vi "FPGA Main_Scripted_OneNode_5-20-2015.vi"() -> ()   [LabVIEW 2014]
uses:
  <vilib>/rvi/Emulation/niFpgaGetClockAttributes.vi
  <vilib>/rvi/Emulation/niFpgaSctlEmulationGetInTimedLoop.vi
  <vilib>/rvi/Emulation/niFpgaEmulationReportErrorSimple.vi
  <vilib>/rvi/Emulation/niFpgaProcessEmulError.vi
  <vilib>/rvi/interface/RandomDataEmulation/niFpgaRandomDataHandleErrors.vi
  <vilib>/rvi/Emulation/niFpgaCriticalErrorInLSC.vi
  <vilib>/rvi/DataTransferAndStorage/Container/XNode/niFpgaContainer.xnode
  <vilib>/rvi/interface/RandomDataEmulation/nirviRandomDataFpgaReadWriteTemplate.vi
  SPIBus0/IO Node Logic Template_SPIBus0.lvlib
panel:
  out "Iteration count":i32
  in  "Debug":bool
  out "FPGA Error":errorcluster
  out "Finished":bool
  in  "stop":bool
  out "Module Underflow":bool
  out "Acq Loop Ticks":u32
  out "DMA FIFO Full":bool
  out "Chan Count":bool
  out "First Read":bool
  in  "Number of Channels":i32=4
  in  "Acquisition Type":enum16{"Finite Samples", "Continuous Samples"}(ring)
  in  "Samps per Chan [Finite]":i32=5120
  in  "Chan Scale Array":sgl[](array[numeric])=[0.0, 0.0, 0.0, 0.0, 0.0, 0.0, 0.0, 0.0, 0.0, 0.0, 0.0, 0.0, 0.0, 0.0, 0.0, 0.0, 0.0, 0.0, 0.0, 0.0, 0.0, 0.0, 0.0, 0.0, 0.0, 0.0, 0.0, 0.0, 0.0, 0.0, 0.0, 0.0, 0.0, 0.0, 0.0, 0.0, 0.0, 0.0, 0.0, 0.0]
  out "oclk mult":u32
  out "oclk div":u32
  out "oclk freq":u32
  in  "data rate (S/s)":u32
  # "Array size fixed at 40\nelements but may be \nexpanded if needed"
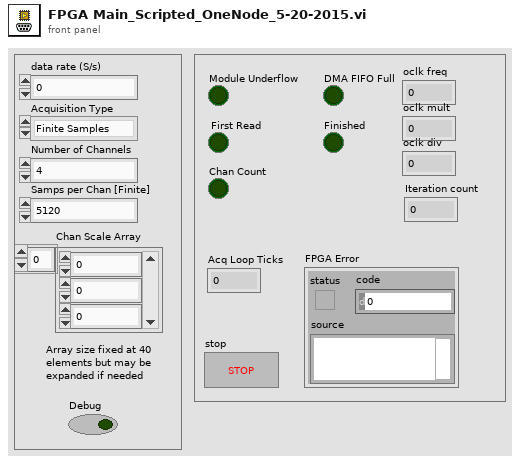
[diagram p1: front panel]
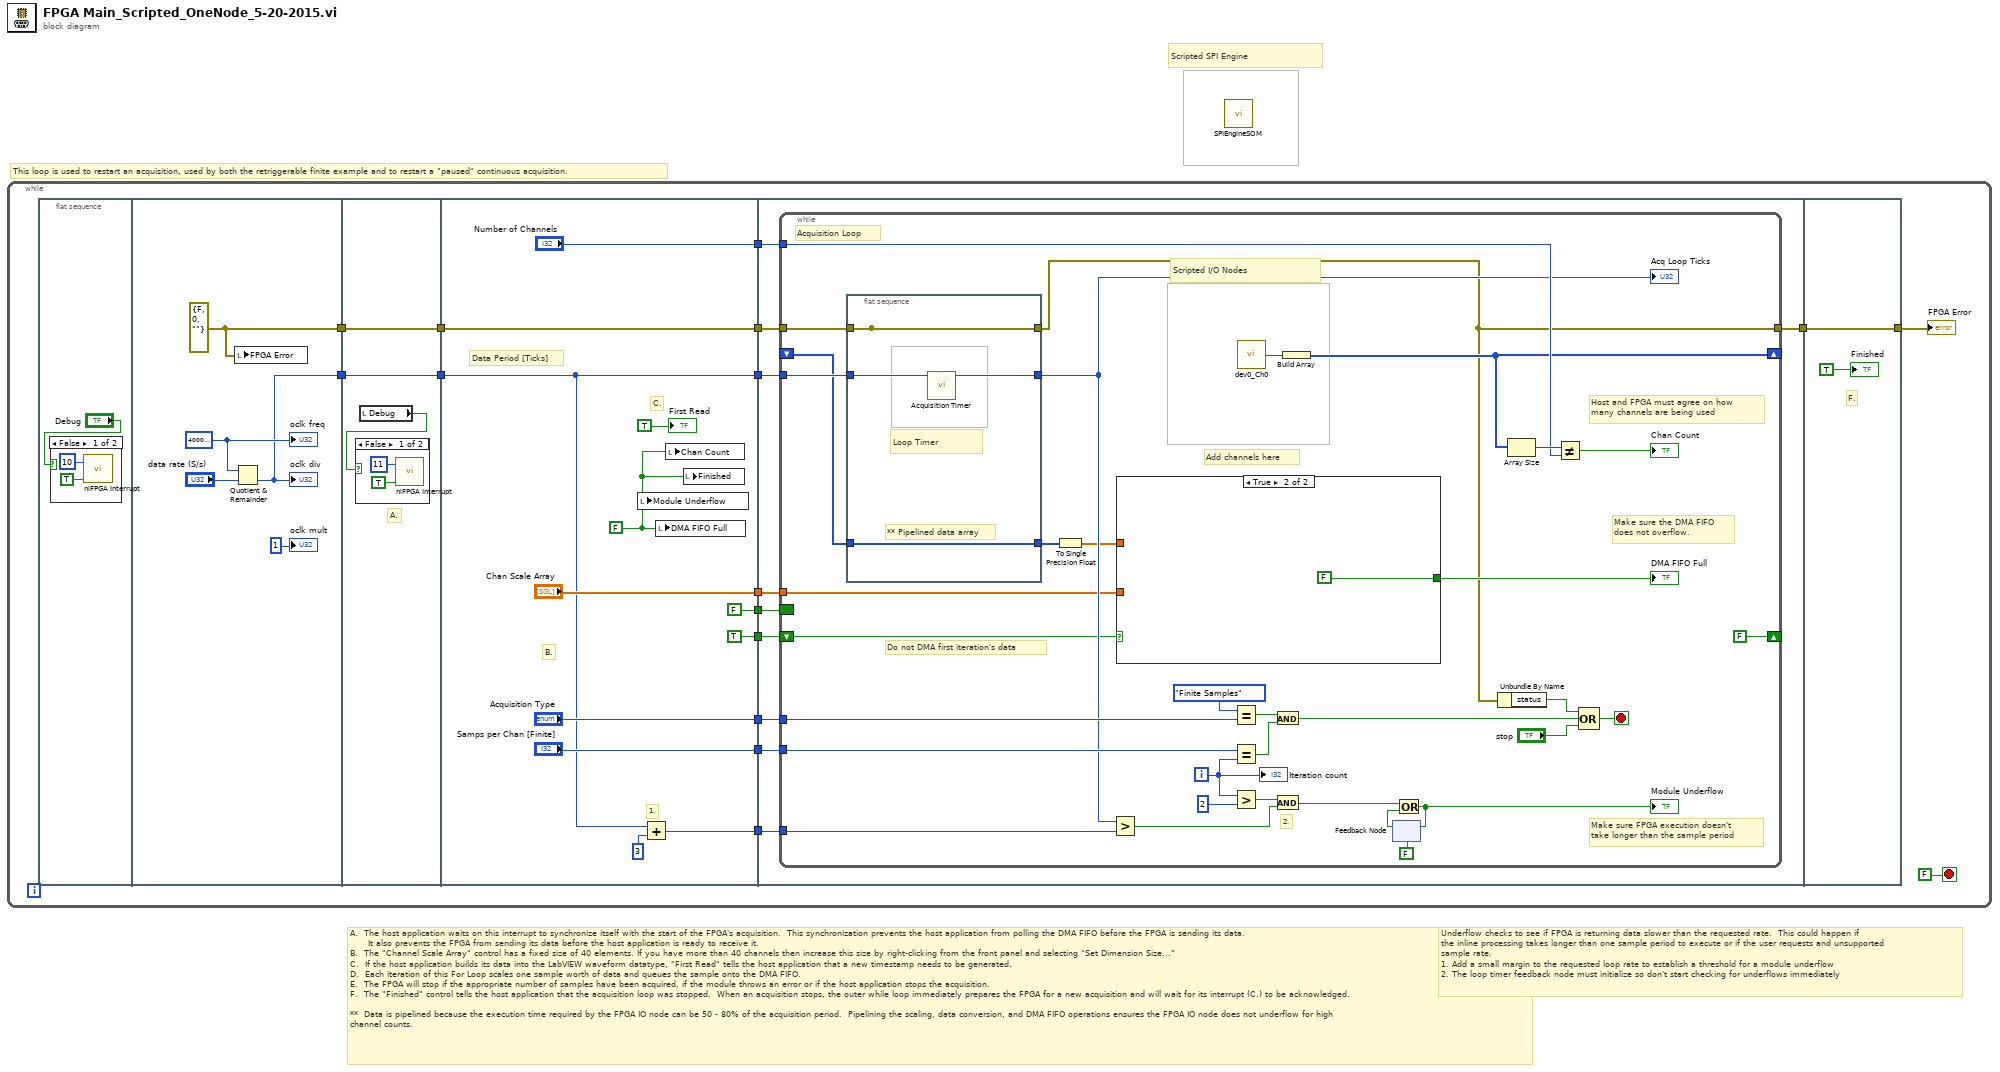
[diagram p0: block diagram]
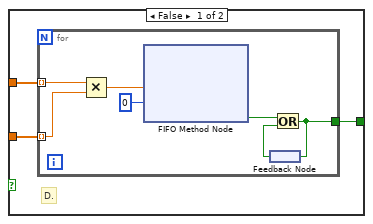
[diagram p4: hidden frame]
diagram:
  # "Scripted SPI Engine"
  # "Underflow checks to see if FPGA is returning data slower than the requested rate.  This could happen if\nthe inline processing takes longer than one sample period to execute or if the user requests and unsupported\nsample rate.\n1. Add a small margin to the requested loop rate to establish a threshold for a module underflow \n2. The loop timer feedback node must initialize so don't start checking for underflows immediately"
  # "A.  The host application waits on this interrupt to synchronize itself with the start of the FPGA's acquisition.  This synchronization prevents the host application from polling the DMA FIFO before the FPGA is sending its data.\n      It also prevents the FPGA from sending its data before the host application is ready to receive it.\nB.  The \"Channel Scale Array\" control has a fixed size of 40 elements. If you have more than 40 channels then increase this size by right-clicking from the front panel and selecting \"Set Dimension Size...\"\nC.  If the host application builds its data into the LabVIEW waveform datatype, \"First Read\" tells the host application that a new timestamp needs to be generated.\nD.  Each iteration of this For Loop scales one sample worth of data and queues the sample onto the DMA FIFO.  \nE.  The FPGA will stop if the appropriate number of samples have been acquired, if the module throws an error or if the host application stops the acquisition.  \nF.  The \"Finished\" control tells the host application that the acquisition loop was stopped.  When an acquisition stops, the outer while loop immediately prepares the FPGA for a new acquisition and will wait for its interrupt (C.) to be acknowledged. \n\n**  Data is pipelined because the execution time required by the FPGA IO node can be 50 - 80% of the acquisition period.  Pipelining the scaling, data conversion, and DMA FIFO operations ensures the FPGA IO node does not underflow for high\nchannel counts."
  # "This loop is used to restart an acquisition, used by both the retriggerable finite example and to restart a \"paused\" continuous acquisition."
  n1 = while {
    stop <- FALSE stop-if-true
    n2 = flat-sequence {
      tunnel: [w21] -> w7
      tunnel: [w20] -> w3
      tunnel: w7 -> [w27]
      tunnel: [w27] -> w6
      tunnel: [w26] -> w4
      tunnel: w3 -> [w26]
      tunnel: ["Number of Channels"] -> w16
      tunnel: ["Chan Scale Array"] -> w15
      tunnel: ["Acquisition Type"] -> w14
      tunnel: ["Samps per Chan [Finite]"] -> w13
      tunnel: [w31] -> w12
      tunnel: [w35] -> w11
      tunnel: [TRUE] -> w10
      tunnel: w6 -> [w32]
      tunnel: [w32] -> w5
      tunnel: w4 -> [w31]
      tunnel: [FALSE] -> w2
      tunnel: w16 -> [w51]
      tunnel: w15 -> [w48]
      tunnel: w14 -> [w47]
      tunnel: w13 -> [w46]
      tunnel: w12 -> [w49]
      tunnel: w11 -> [w45]
      tunnel: w10 -> [w44]
      tunnel: [w43] -> w8
      tunnel: w5 -> [w50]
      tunnel: w2 -> [w42]
      tunnel: [w101] -> w9
      tunnel: w8 -> [w101]
      frame #0 {
        n3 = case shown="False" "Debug" {
          frame False {
            n4 = call <vilib>:"niFPGA Interrupt.vi"("Wait Until Cleared (F)"=TRUE ("Wait Until Cleared"), "IRQ Number (0)"=u8 10 ("IRQ Number")) -> ()  [unwired: 1 in]
          }
          frame True {
          }
        }
      }
      frame #1 {
        w21 = errorcluster {"status"=FALSE, "code"=0, "source"=""} ("FPGA Error")
        w22 = u32 40000000 ("oclk freq")
        n5 = Quotient & Remainder(x=w22, y="data rate (S/s)") -> (floor(x/y)=w20:u32)  [unwired: 1 out]
        "oclk div" <- w20
        n6 = local write "FPGA Error"(w21) -> ()
        "oclk mult" <- u32 1 ("oclk mult")
        "oclk freq" <- w22
      }
      frame #2 {
        # "A."
        n7 = local read "Debug"() -> (w25:bool)
        n8 = case shown="False" w25 {
          frame False {
            n9 = call <vilib>:"niFPGA Interrupt.vi"("Wait Until Cleared (F)"=TRUE ("Wait Until Cleared"), "IRQ Number (0)"=u8 11 ("IRQ Number")) -> ()  [unwired: 1 in]
          }
          frame True {
          }
        }
      }
      frame #3 {
        w40 = FALSE ("Module Underflow")
        # "Data Period [Ticks]"
        # "1."
        # "C."
        # "B."
        n10 = local write "Module Underflow"(w40) -> ()
        n11 = Add(x=w31, y=u32 3) -> (x+y=w35:u32)
        n12 = local write "DMA FIFO Full"(w40) -> ()
        n13 = local write "Chan Count"(w40) -> ()
        n14 = local write "Finished"(w40) -> ()
        "First Read" <- TRUE ("First Read")
      }
      frame #4 {
        n15 = while {
          tunnel: w47 -> [w78]
          tunnel: w46 -> [w77]
          shift-right: [w56] -> _
          shift-left: _ -> [w69]
          tunnel: w51 -> [w79]
          tunnel: w50 -> [w71]
          tunnel: [w53] -> w43
          tunnel: w49 -> [w76]
          tunnel: w45 -> [w72]
          tunnel: w48 -> [w68]
          shift-right: [FALSE] -> _
          shift-left: w44 -> [w67]
          border: w42 -> [_]
          i -> [w65]
          stop <- w83 stop-if-true
          # "Scripted I/O Nodes"
          # "Add channels here"
          # "2."
          # "Do not DMA first iteration's data"
          # "Host and FPGA must agree on how \nmany channels are being used"
          # "Acquisition Loop"
          # "Make sure the DMA FIFO\ndoes not overflow."
          # "Make sure FPGA execution doesn't\ntake longer than the sample period"
          n16 = flat-sequence {
            tunnel: w76 -> [w99]
            tunnel: [w97] -> _
            tunnel: w71 -> [w97]
            tunnel: [w98] -> w70
            tunnel: [w100] -> w55
            tunnel: w69 -> [w100]
            tunnel: [w97] -> w53
            frame #0 {
              # "Loop Timer"
              # "** Pipelined data array"
              n17 = call <vilib>:"Acquisition Timer.vi"("Loop Time (Ticks)"=w99) -> ("Actual Time (Ticks)"=w98:u32)  [unwired: 10 in]
            }
          }
          n18 = To Single Precision Float(number=w55) -> (single precision float=w54:sgl[])
          n19 = Greater?(x=w70, y=w72) -> (0:w75:bool)
          n20 = case shown="True" w67 {
            tunnel: [w88 FALSE] -> w82
            tunnel: w54 -> [w87 _]
            tunnel: w68 -> [w86 _]
            frame False {
              # "D."
              n21 = for {
                tunnel: [w94] -> w88
                tunnel: w87 -> [w93] mode=indexing
                tunnel: w86 -> [w89] mode=indexing
                n22 = Multiply(x=w93, y=w89) -> (x*y=w90:sgl)
                n23 = xnode ("FIFO Method Node")("Element"=w90, "Timeout"=0) -> ("Timed Out?"=w91:bool)  [unwired: 1 in, 1 out]
                n24 = feedback #1() -> (w95:bool)
                n25 = Or(x=w91, y=w95) -> (x .or. y?=w94:bool)
                n26 = feedback-in #1(w94) -> ()
              }
            }
            frame True {
            }
          }
          "DMA FIFO Full" <- w82
          n27 = Equal?(x=enum16{"Finite Samples", "Continuous Samples"}."Finite Samples" ("y"), y=w78) -> (x = y?=w59:bool)
          n28 = Equal?(x=w77, y=w65) -> (x = y?=w58:bool)
          n29 = Greater?(x=w65, y=2) -> (0:w74:bool)
          n30 = call "dev0_Ch0.vi"() -> ("Received Data"=w52:u64)  [unwired: 15 in]
          n31 = And(x=w59, y=w58) -> (x .and. y?=w57:bool)
          n32 = And(x=w74, y=w75) -> (x .and. y?=w61:bool)
          n33 = Build Array(w52) -> (w56:u64[])
          n34 = feedback #2(FALSE) -> (w63:bool)
          n35 = Or(x=w61, y=w63) -> (x .or. y?=w60:bool)
          "Module Underflow" <- w60
          n36 = feedback-in #2(w60) -> ()
          n37 = Unbundle By Name(w53) -> ("status"=w64:bool)
          n38 = Array Size(array=w56) -> (size(s)=w81:i32)
          n39 = Not Equal?(x=w81, y=w79) -> (x != y?=→"Chan Count":bool)
          n40 = Compound Arithmetic op=OR(w64, w57, "stop") -> (w83:bool)
          "Acq Loop Ticks" <- w70
          "Iteration count" <- w65
        }
      }
      frame #5 {
        # "F."
        "Finished" <- TRUE ("Finished")
      }
    }
    "FPGA Error" <- w9
  }
  n41 = call "SPIEngineSOM.vi"() -> ()  [unwired: 12 in]
